vi "SmoothLine.vi"(8 "error in (no error)":errorcluster, 9 "Parameters":T2={"number of planes"=4, "z step"=1.9999999999999998e-05, "pixel dwell time"=1.0000000000000001e-11, "z frequency"=10.0, "number of pixels"=100, "smooth points"=10, "smooth line"=10, "Sine\nSawtooth"=FALSE, "PointSorting"=0, "Sort Points"=FALSE, "X-pixels"=256.0, "Y-lines"=256.0, "pixelstoµm"=256.0, "zoom"=1.0, "Time offset"=1.0000000000000001e-11} {"zoom" min=0.5 step=0.1; "Y-lines" min=1 step=1; "X-pixels" min=1 step=1; "PointSorting" items=["No Difference", "Every Second Point", "Down / Up"]; "smooth line" min=1; "smooth points" min=1; "number of pixels" min=1; "z frequency" format="%_4g"; "number of planes" min=1}, 10 "DutyCluster":T1 {"Iteration" items=["first iteration", "second iteration"]}, 11 "XYZ Point coordinates (pixels)":dbl[][](array[numeric])) -> (0 "error out":errorcluster, 2 "DutyCluster":T1 {"Iteration" items=["first iteration", "second iteration"]}, 3 "XYZ Point coordinates smoothed (pixels)":dbl[][](array[numeric]))   [LabVIEW 2010]
uses:
  TypeDefs/DutyCluster.ctl
  TypeDefs/ParameterCluster.ctl
  <vilib>/Analysis/_algsub.llb/Real Vector Norm.vi
  <vilib>/Analysis/NI_AALPro.lvlib
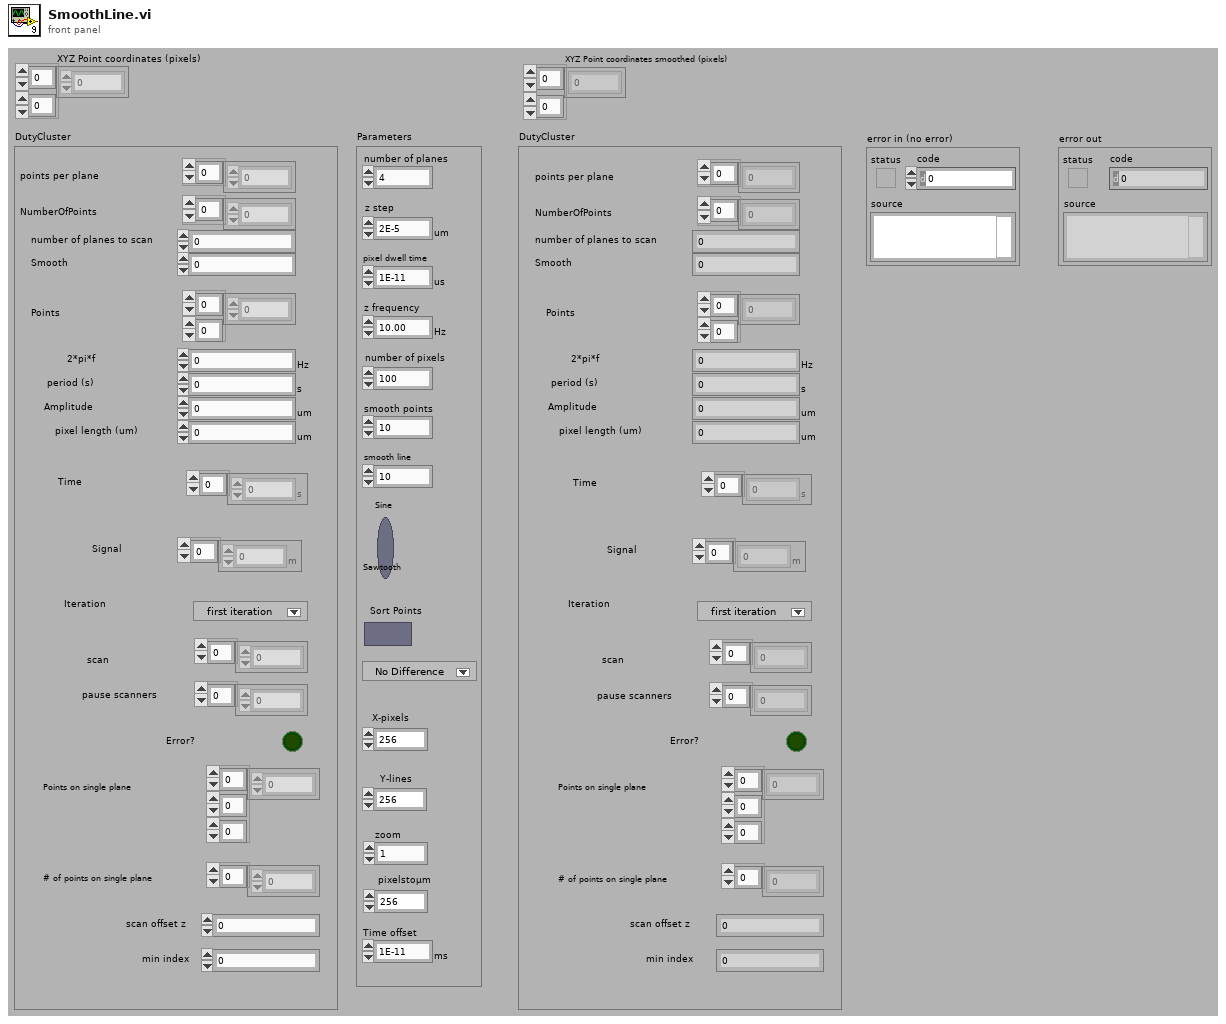
[diagram p1: front panel]
types:
  T1 = typedef "DutyCluster.ctl" = cluster{"points per plane":i32[], "NumberOfPoints":i32[], "number of planes to scan":i32, "Smooth":i32, "Points":dbl[][], "2*pi*f":dbl[unit], "period (s)":dbl[unit], "Amplitude":dbl[unit], "pixel length (um)":dbl[unit], "Time":dbl[unit][], "Signal":dbl[unit][], "Iteration":u16, "scan":i32[], "pause scanners":i32[], "Error?":bool, "Points on single plane":dbl[][][], "# of points on single plane":i32[], "scan offset z":i32, "min index":i32}
  T2 = typedef "ParameterCluster.ctl" = cluster{"number of planes":i32, "z step":dbl[unit], "pixel dwell time":dbl[unit], "z frequency":dbl[unit], "number of pixels":i32, "smooth points":i32, "smooth line":i32, "Sine\nSawtooth":bool, "PointSorting":u16, "Sort Points":bool, "X-pixels":sgl, "Y-lines":sgl, "pixelstoµm":dbl, "zoom":dbl, "Time offset":dbl[unit]}
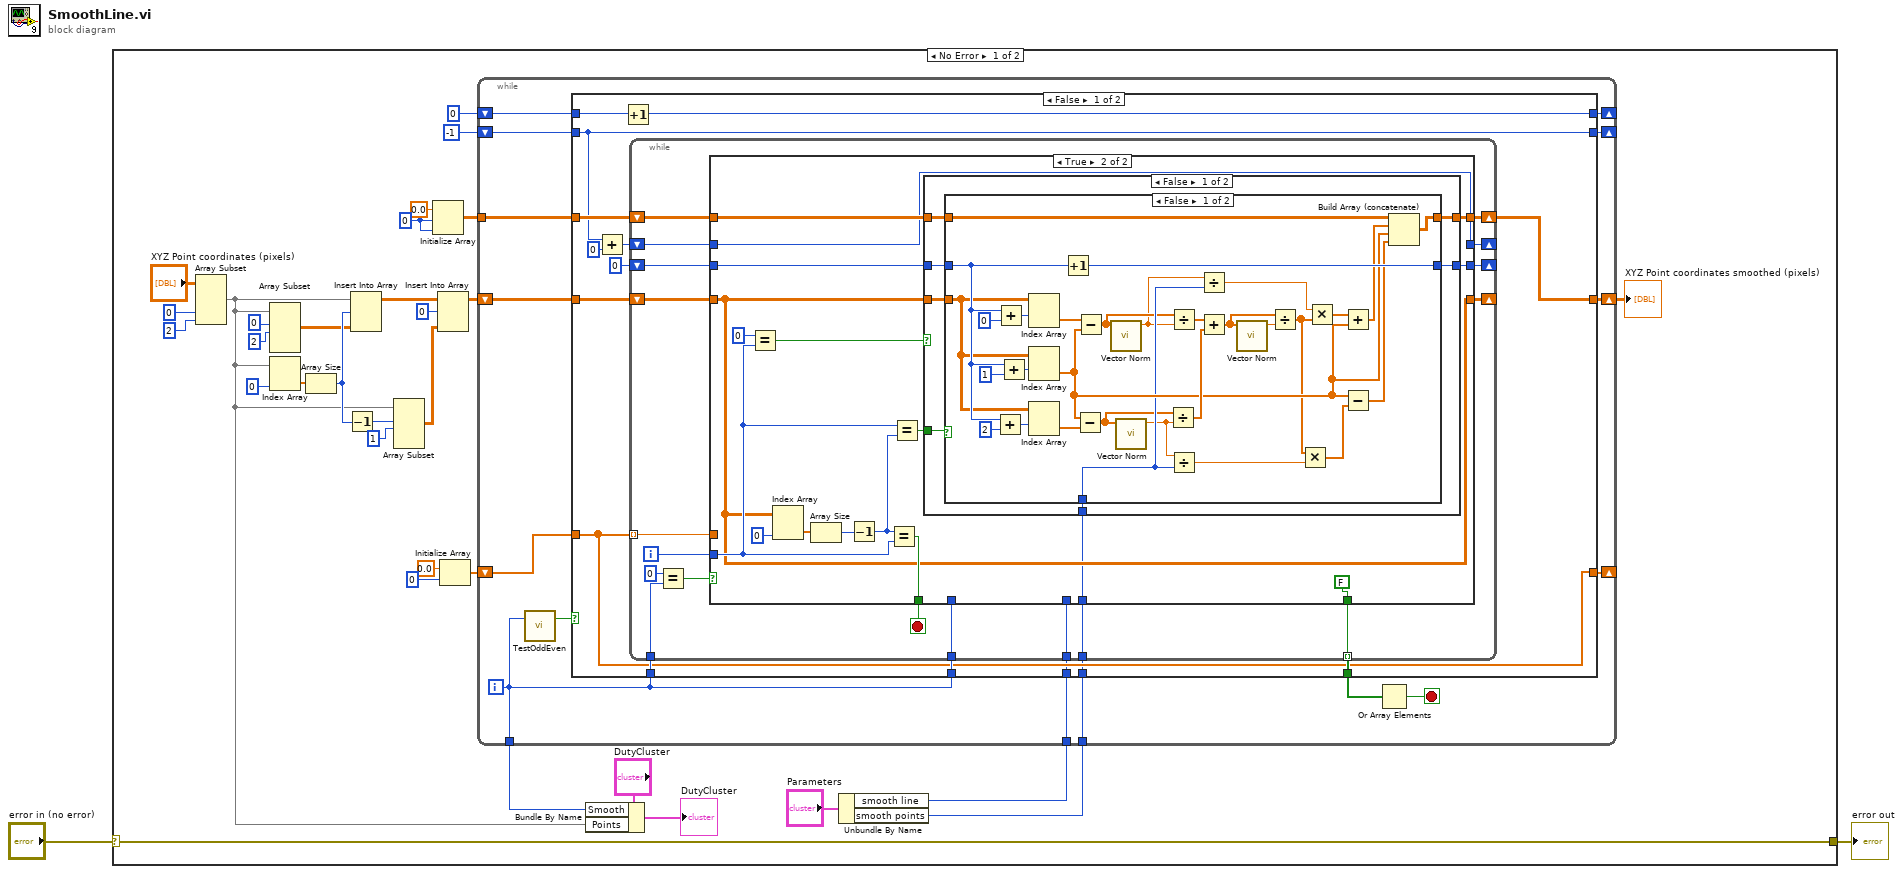
[diagram p0: block diagram]
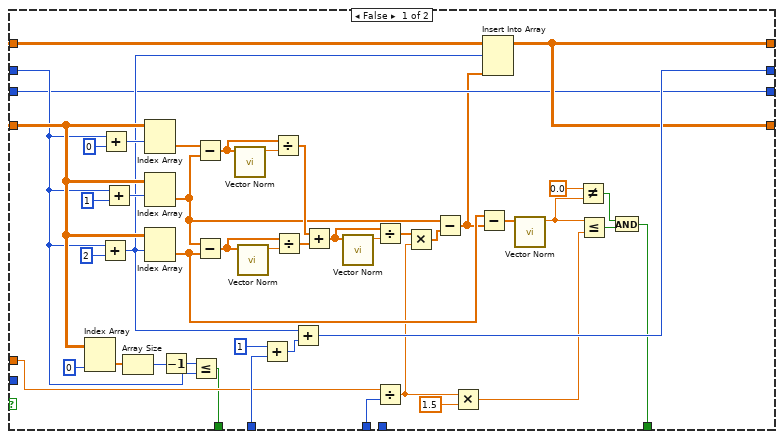
[diagram p2: hidden frame]
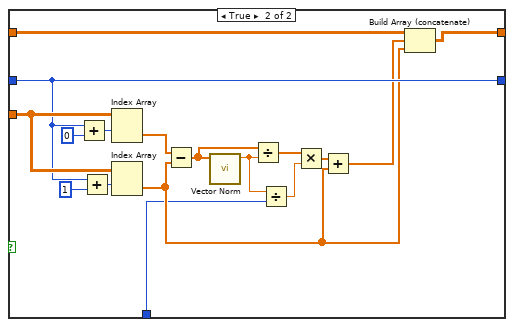
[diagram p3: hidden frame]
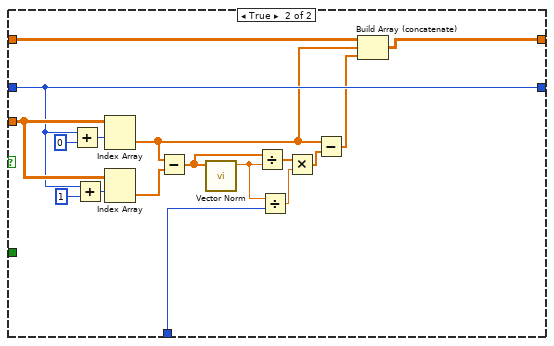
[diagram p4: hidden frame]
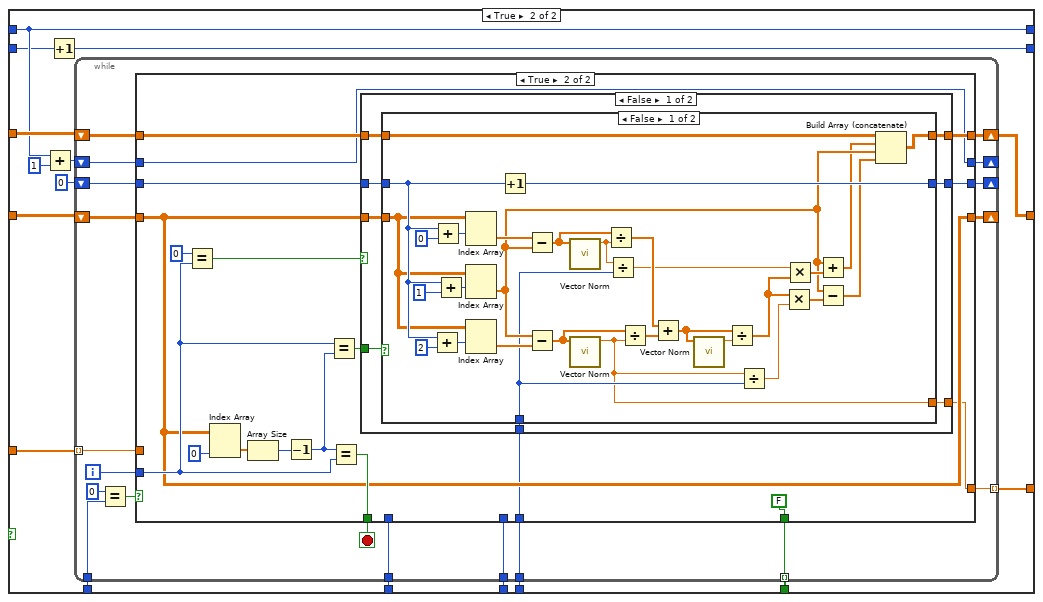
[diagram p5: hidden frame]
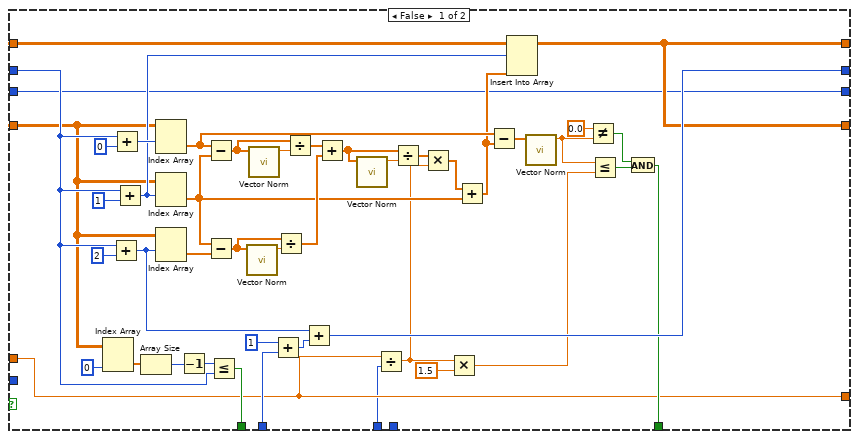
[diagram p6: hidden frame]
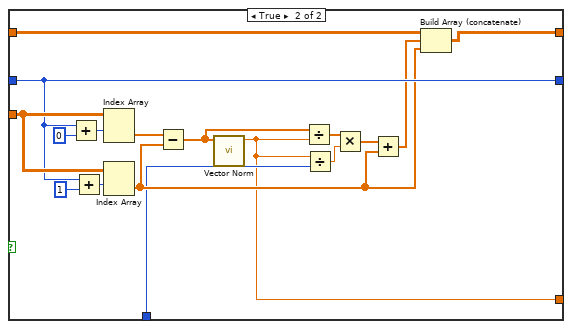
[diagram p7: hidden frame]
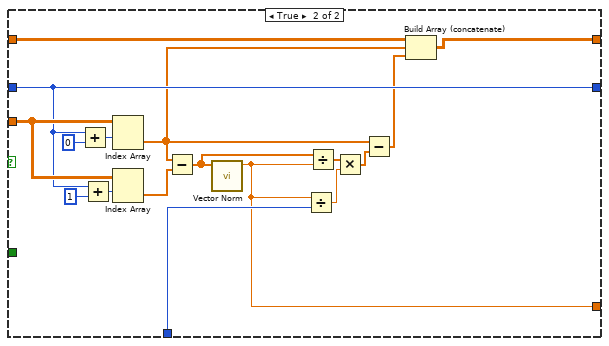
[diagram p8: hidden frame]
diagram:
  n1 = case shown="No Error" "error in (no error)" {
    selector: "error in (no error)" -> [w5 w384]
    tunnel: [w5 w384] -> w1
    frame No Error {
      w10 = 0 ("dimension size")
      n2 = Array Subset(array="XYZ Point coordinates (pixels)", index (col)=0 ("index"), length (col)=2 ("length")) -> (w9:dbl[][])  [unwired: 2 in]
      n3 = Array Subset(array=w9, index (row)=0 ("disabled index (col)"), length (row)=2 ("length")) -> (w17:dbl[][])  [unwired: 2 in]
      n4 = Index Array(array=w9, index (col)=0 ("disabled index (col)")) -> (element=w15:dbl[])  [unwired: 1 in]
      n5 = Array Size(array=w15) -> (size(s)=w18:i32)
      n6 = Decrement(x=w18) -> (x-1=w24:i32)
      n7 = Insert Into Array(array=w9, index (row)=w18, new element=w17) -> (w21:dbl[][])  [unwired: 1 in]
      n8 = Array Subset(array=w9, index (row)=w24, length (row)=1 ("length")) -> (w19:dbl[][])  [unwired: 2 in]
      n9 = Initialize Array(0.0 ("element"), w10, w10) -> (w33:dbl[][])
      n10 = Insert Into Array(array=w21, index (row)=0, new element=w19) -> (w27:dbl[][])  [unwired: 1 in]
      n11 = Initialize Array(0.0 ("element"), 0 ("dimension size")) -> (w28:dbl[])
      n12 = Unbundle By Name("Parameters") -> ("smooth line"=w8:i32, "smooth points"=w7:i32)
      n13 = while {
        shift-right: [w47] -> w6
        shift-left: w27 -> [w49]
        tunnel: w33 -> [w48]
        shift-right: [w43] -> _
        shift-left: 0 ("index") -> [w44]
        shift-right: [w41] -> _
        shift-left: -1 ("index") -> [w42]
        tunnel: [w40] -> w12
        shift-right: [w39] -> _
        shift-left: w28 -> [w38]
        tunnel: w8 -> [w36]
        tunnel: w7 -> [w35]
        i -> [w40]
        stop <- w37 stop-if-true
        n14 = call "TestOddEven.vi"("Numeric"=w40) -> ("Boolean"=w45:bool)  [unwired: 1 in, 1 out]
        n15 = case shown="False" w45 {
          tunnel: w49 -> [w63 w229]
          tunnel: w48 -> [w62 w230]
          tunnel: [w61 w224] -> w47
          tunnel: [w60 w228] -> w46
          tunnel: w40 -> [w59 w227]
          tunnel: w40 -> [w58 w226]
          tunnel: w44 -> [w57 w221]
          tunnel: [w56 w221] -> w43
          tunnel: w42 -> [w55 w220]
          tunnel: [w55 w219] -> w41
          tunnel: [w52 w218] -> w39
          tunnel: w38 -> [w52 w217]
          tunnel: w36 -> [w51 w216]
          tunnel: w35 -> [w50 w215]
          frame False {
            n16 = Add(x=w55, y=0) -> (x+y=w54:i32)
            n17 = Increment(x=w57) -> (x+1=w56:i32)
            n18 = while {
              shift-right: [w82] -> _
              shift-left: 0 ("index") -> [w78]
              shift-right: [w80] -> w61
              shift-left: w62 -> [w81]
              tunnel: w59 -> [w71]
              shift-right: [w75] -> _
              shift-left: w54 -> [w70]
              shift-right: [w74] -> _
              shift-left: w63 -> [w79]
              tunnel: w58 -> [w73]
              tunnel: [w72] -> w60 mode=indexing
              tunnel: w52 -> [w68] mode=indexing
              tunnel: w51 -> [w66]
              tunnel: w50 -> [w65]
              i -> [w69]
              stop <- w67 stop-if-true
              n19 = Equal?(x=0 ("y"), y=w71) -> (x = y?=w76:bool)
              n20 = case shown="True" w76 {
                tunnel: [w99 w143] -> w82
                tunnel: [w92 w142] -> w67
                tunnel: w81 -> [_ w141]
                tunnel: [w115 w140] -> w80
                tunnel: w79 -> [w105 w129]
                tunnel: w78 -> [w99 w137]
                tunnel: w69 -> [_ w133]
                tunnel: w70 -> [w101 w130]
                tunnel: [w116 w130] -> w75
                tunnel: [w115 w129] -> w74
                tunnel: w73 -> [w111 _]
                tunnel: [w109 FALSE] -> w72
                tunnel: w68 -> [w94 _]
                tunnel: w66 -> [w91 _]
                tunnel: w65 -> [_ w127]
                frame False {
                  n21 = Index Array(array=w105, index (col)=0 ("disabled index (col)")) -> (element=w126:dbl[])  [unwired: 1 in]
                  n22 = Add(x=w101, y=2 ("disabled index (col)")) -> (x+y=w104:i32)
                  n23 = Add(x=w101, y=0 ("disabled index (col)")) -> (x+y=w121:i32)
                  n24 = Add(x=w101, y=1 ("disabled index (col)")) -> (x+y=w114:i32)
                  n25 = Array Size(array=w126) -> (size(s)=w124:i32)
                  n26 = Index Array(array=w105, index (row)=w121) -> (element=w108:dbl[])  [unwired: 1 in]
                  n27 = Index Array(array=w105, index (row)=w114) -> (element=w102:dbl[])  [unwired: 1 in]
                  n28 = Index Array(array=w105, index (row)=w104) -> (element=w100:dbl[])  [unwired: 1 in]
                  n29 = Decrement(x=w124) -> (x-1=w123:i32)
                  n30 = Less Or Equal?(x=w123, y=w101) -> (x <= y?=w92:bool)
                  n31 = Subtract(x=w108, y=w102) -> (x-y=w90:dbl[])
                  n32 = Subtract(x=w102, y=w100) -> (x-y=w88:dbl[])
                  n33 = call-poly <vilib>:"Vector Norm.vi"("Input Vector"=w90) -> ("norm"=w89:dbl)  [unwired: 9 in, 1 out]
                  n34 = call-poly <vilib>:"Vector Norm.vi"("Input Vector"=w88) -> ("norm"=w87:dbl)  [unwired: 9 in, 1 out]
                  n35 = Add(x=1 ("y"), y=w111) -> (x+y=w113:i32)
                  n36 = Divide(x=w90, y=w89) -> (x/y=w118:dbl[])
                  n37 = Divide(x=w88, y=w87) -> (x/y=w117:dbl[])
                  n38 = Add(x=w104, y=w113) -> (x+y=w116:i32)
                  n39 = Add(x=w118, y=w117) -> (x+y=w86:dbl[])
                  n40 = call-poly <vilib>:"Vector Norm.vi"("Input Vector"=w86) -> ("norm"=w85:dbl)  [unwired: 9 in, 1 out]
                  n41 = Divide(x=w86, y=w85) -> (x/y=w97:dbl[])
                  n42 = Divide(x=w94, y=w91) -> (x/y=w93:dbl)
                  n43 = Multiply(x=w97, y=w93) -> (x*y=w103:dbl[])
                  n44 = Subtract(x=w102, y=w103) -> (x-y=w98:dbl[])
                  n45 = Multiply(x=w93, y=1.5) -> (x*y=w95:dbl)
                  n46 = Subtract(x=w100, y=w98) -> (x-y=w84:dbl[])
                  n47 = Insert Into Array(array=w105, index (row)=w104, new element=w98) -> (w115:dbl[][])  [unwired: 1 in]
                  n48 = call-poly <vilib>:"Vector Norm.vi"("Input Vector"=w84) -> ("norm"=w83:dbl)  [unwired: 9 in, 1 out]
                  n49 = Not Equal?(x=0.0, y=w83) -> (x != y?=w107:bool)
                  n50 = Less Or Equal?(x=w83, y=w95) -> (x <= y?=w110:bool)
                  n51 = And(x=w107, y=w110) -> (x .and. y?=w109:bool)
                }
                frame True {
                  n52 = Equal?(x=0 ("y"), y=w133) -> (x = y?=w136:bool)
                  n53 = Index Array(array=w129, index (col)=0 ("disabled index (col)")) -> (element=w139:dbl[])  [unwired: 1 in]
                  n54 = Array Size(array=w139) -> (size(s)=w132:i32)
                  n55 = Decrement(x=w132) -> (x-1=w131:i32)
                  n56 = Equal?(x=w131, y=w133) -> (x = y?=w142:bool)
                  n57 = Equal?(x=w133, y=w131) -> (x = y?=w134:bool)
                  n58 = case shown="False" w136 {
                    tunnel: [w150 w211] -> w143
                    tunnel: w137 -> [w149 w211]
                    tunnel: w141 -> [w148 w213]
                    tunnel: [w147 w212] -> w140
                    tunnel: w129 -> [w146 w214]
                    tunnel: w134 -> [w145 _]
                    tunnel: w127 -> [w144 w200]
                    frame False {
                      n59 = case shown="False" w145 {
                        tunnel: [w174 w189] -> w150
                        tunnel: w149 -> [w173 w189]
                        tunnel: w148 -> [w172 w192]
                        tunnel: [w166 w191] -> w147
                        tunnel: w146 -> [w165 w190]
                        tunnel: w144 -> [w157 w183]
                        frame False {
                          n60 = Add(x=w173, y=2 ("disabled index (col)")) -> (x+y=w175:i32)
                          n61 = Add(x=w173, y=0 ("disabled index (col)")) -> (x+y=w179:i32)
                          n62 = Add(x=w173, y=1 ("disabled index (col)")) -> (x+y=w177:i32)
                          n63 = Index Array(array=w165, index (row)=w179) -> (element=w170:dbl[])  [unwired: 1 in]
                          n64 = Index Array(array=w165, index (row)=w177) -> (element=w164:dbl[])  [unwired: 1 in]
                          n65 = Index Array(array=w165, index (row)=w175) -> (element=w171:dbl[])  [unwired: 1 in]
                          n66 = Increment(x=w173) -> (x+1=w174:i32)
                          n67 = Subtract(x=w164, y=w171) -> (x-y=w154:dbl[])
                          n68 = Subtract(x=w170, y=w164) -> (x-y=w156:dbl[])
                          n69 = call-poly <vilib>:"Vector Norm.vi"("Input Vector"=w156) -> ("norm"=w155:dbl)  [unwired: 9 in, 1 out]
                          n70 = call-poly <vilib>:"Vector Norm.vi"("Input Vector"=w154) -> ("norm"=w153:dbl)  [unwired: 9 in, 1 out]
                          n71 = Divide(x=w154, y=w153) -> (x/y=w168:dbl[])
                          n72 = Divide(x=w156, y=w155) -> (x/y=w169:dbl[])
                          n73 = Divide(x=w153, y=w157) -> (x/y=w159:dbl)
                          n74 = Divide(x=w155, y=w157) -> (x/y=w158:dbl)
                          n75 = Add(x=w169, y=w168) -> (x+y=w152:dbl[])
                          n76 = call-poly <vilib>:"Vector Norm.vi"("Input Vector"=w152) -> ("norm"=w151:dbl)  [unwired: 9 in, 1 out]
                          n77 = Divide(x=w152, y=w151) -> (x/y=w161:dbl[])
                          n78 = Multiply(x=w161, y=w159) -> (x*y=w160:dbl[])
                          n79 = Multiply(x=w158, y=w161) -> (x*y=w167:dbl[])
                          n80 = Add(x=w167, y=w164) -> (x+y=w162:dbl[])
                          n81 = Subtract(x=w164, y=w160) -> (x-y=w163:dbl[])
                          n82 = Build Array (concatenate)(w172, w162, w164, w163) -> (w166:dbl[][])
                        }
                        frame True {
                          n83 = Add(x=w189, y=0 ("disabled index (col)")) -> (x+y=w196:i32)
                          n84 = Add(x=w189, y=1 ("disabled index (col)")) -> (x+y=w194:i32)
                          n85 = Index Array(array=w190, index (row)=w196) -> (element=w193:dbl[])  [unwired: 1 in]
                          n86 = Index Array(array=w190, index (row)=w194) -> (element=w187:dbl[])  [unwired: 1 in]
                          n87 = Subtract(x=w193, y=w187) -> (x-y=w182:dbl[])
                          n88 = call-poly <vilib>:"Vector Norm.vi"("Input Vector"=w182) -> ("norm"=w181:dbl)  [unwired: 9 in, 1 out]
                          n89 = Divide(x=w182, y=w181) -> (x/y=w185:dbl[])
                          n90 = Divide(x=w181, y=w183) -> (x/y=w184:dbl)
                          n91 = Multiply(x=w185, y=w184) -> (x*y=w188:dbl[])
                          n92 = Add(x=w188, y=w187) -> (x+y=w186:dbl[])
                          n93 = Build Array (concatenate)(w192, w186, w187) -> (w191:dbl[][])
                        }
                      }
                    }
                    frame True {
                      n94 = Add(x=w211, y=0 ("disabled index (col)")) -> (x+y=w209:i32)
                      n95 = Add(x=w211, y=1 ("disabled index (col)")) -> (x+y=w207:i32)
                      n96 = Index Array(array=w214, index (row)=w209) -> (element=w206:dbl[])  [unwired: 1 in]
                      n97 = Index Array(array=w214, index (row)=w207) -> (element=w205:dbl[])  [unwired: 1 in]
                      n98 = Subtract(x=w206, y=w205) -> (x-y=w199:dbl[])
                      n99 = call-poly <vilib>:"Vector Norm.vi"("Input Vector"=w199) -> ("norm"=w198:dbl)  [unwired: 9 in, 1 out]
                      n100 = Divide(x=w199, y=w198) -> (x/y=w203:dbl[])
                      n101 = Divide(x=w198, y=w200) -> (x/y=w201:dbl)
                      n102 = Multiply(x=w203, y=w201) -> (x*y=w204:dbl[])
                      n103 = Subtract(x=w206, y=w204) -> (x-y=w202:dbl[])
                      n104 = Build Array (concatenate)(w213, w206, w202) -> (w212:dbl[][])
                    }
                  }
                }
              }
            }
          }
          frame True {
            n105 = Add(x=w221, y=1 ("index")) -> (x+y=w222:i32)
            n106 = Increment(x=w220) -> (x+1=w219:i32)
            n107 = while {
              shift-right: [w249] -> _
              shift-left: 0 ("index") -> [w245]
              shift-right: [w247] -> w224
              shift-left: w230 -> [w248]
              tunnel: w227 -> [w242]
              shift-right: [w239] -> _
              shift-left: w222 -> [w240]
              shift-right: [w238] -> _
              shift-left: w229 -> [w246]
              tunnel: w226 -> [w237]
              tunnel: [w236] -> w228 mode=indexing
              tunnel: [w235] -> w218 mode=indexing
              tunnel: w217 -> [w234] mode=indexing
              tunnel: w216 -> [w232]
              tunnel: w215 -> [w231]
              i -> [w244]
              stop <- w233 stop-if-true
              n108 = Equal?(x=0 ("y"), y=w242) -> (x = y?=w241:bool)
              n109 = case shown="True" w241 {
                tunnel: [w264 w311] -> w249
                tunnel: [w290 w310] -> w233
                tunnel: w248 -> [_ w309]
                tunnel: [w279 w308] -> w247
                tunnel: w246 -> [w268 w297]
                tunnel: w245 -> [w264 w305]
                tunnel: w244 -> [_ w301]
                tunnel: w240 -> [w281 w298]
                tunnel: [w280 w298] -> w239
                tunnel: [w279 w297] -> w238
                tunnel: w237 -> [w274 _]
                tunnel: [w272 FALSE] -> w236
                tunnel: [w260 w295] -> w235
                tunnel: w234 -> [w260 _]
                tunnel: w232 -> [w258 _]
                tunnel: w231 -> [_ w294]
                frame False {
                  n110 = Index Array(array=w268, index (col)=0 ("disabled index (col)")) -> (element=w293:dbl[])  [unwired: 1 in]
                  n111 = Add(x=w281, y=2 ("disabled index (col)")) -> (x+y=w277:i32)
                  n112 = Add(x=w281, y=0 ("disabled index (col)")) -> (x+y=w287:i32)
                  n113 = Add(x=w281, y=1 ("disabled index (col)")) -> (x+y=w278:i32)
                  n114 = Array Size(array=w293) -> (size(s)=w291:i32)
                  n115 = Index Array(array=w268, index (row)=w287) -> (element=w271:dbl[])  [unwired: 1 in]
                  n116 = Index Array(array=w268, index (row)=w278) -> (element=w265:dbl[])  [unwired: 1 in]
                  n117 = Index Array(array=w268, index (row)=w277) -> (element=w284:dbl[])  [unwired: 1 in]
                  n118 = Decrement(x=w291) -> (x-1=w289:i32)
                  n119 = Subtract(x=w271, y=w265) -> (x-y=w255:dbl[])
                  n120 = Subtract(x=w265, y=w284) -> (x-y=w257:dbl[])
                  n121 = Less Or Equal?(x=w289, y=w281) -> (x <= y?=w290:bool)
                  n122 = call-poly <vilib>:"Vector Norm.vi"("Input Vector"=w257) -> ("norm"=w256:dbl)  [unwired: 9 in, 1 out]
                  n123 = call-poly <vilib>:"Vector Norm.vi"("Input Vector"=w255) -> ("norm"=w254:dbl)  [unwired: 9 in, 1 out]
                  n124 = Add(x=1 ("y"), y=w274) -> (x+y=w276:i32)
                  n125 = Divide(x=w257, y=w256) -> (x/y=w282:dbl[])
                  n126 = Divide(x=w255, y=w254) -> (x/y=w283:dbl[])
                  n127 = Add(x=w277, y=w276) -> (x+y=w280:i32)
                  n128 = Add(x=w283, y=w282) -> (x+y=w253:dbl[])
                  n129 = call-poly <vilib>:"Vector Norm.vi"("Input Vector"=w253) -> ("norm"=w252:dbl)  [unwired: 9 in, 1 out]
                  n130 = Divide(x=w260, y=w258) -> (x/y=w259:dbl)
                  n131 = Divide(x=w253, y=w252) -> (x/y=w263:dbl[])
                  n132 = Multiply(x=w263, y=w259) -> (x*y=w266:dbl[])
                  n133 = Multiply(x=w259, y=1.5) -> (x*y=w261:dbl)
                  n134 = Add(x=w266, y=w265) -> (x+y=w267:dbl[])
                  n135 = Subtract(x=w271, y=w267) -> (x-y=w251:dbl[])
                  n136 = Insert Into Array(array=w268, index (row)=w278, new element=w267) -> (w279:dbl[][])  [unwired: 1 in]
                  n137 = call-poly <vilib>:"Vector Norm.vi"("Input Vector"=w251) -> ("norm"=w250:dbl)  [unwired: 9 in, 1 out]
                  n138 = Not Equal?(x=0.0, y=w250) -> (x != y?=w270:bool)
                  n139 = Less Or Equal?(x=w250, y=w261) -> (x <= y?=w273:bool)
                  n140 = And(x=w270, y=w273) -> (x .and. y?=w272:bool)
                }
                frame True {
                  n141 = Equal?(x=0 ("y"), y=w301) -> (x = y?=w304:bool)
                  n142 = Index Array(array=w297, index (col)=0 ("disabled index (col)")) -> (element=w307:dbl[])  [unwired: 1 in]
                  n143 = Array Size(array=w307) -> (size(s)=w300:i32)
                  n144 = Decrement(x=w300) -> (x-1=w299:i32)
                  n145 = Equal?(x=w301, y=w299) -> (x = y?=w302:bool)
                  n146 = Equal?(x=w299, y=w301) -> (x = y?=w310:bool)
                  n147 = case shown="False" w304 {
                    tunnel: [w319 w380] -> w311
                    tunnel: w305 -> [w318 w380]
                    tunnel: w309 -> [w317 w382]
                    tunnel: [w316 w381] -> w308
                    tunnel: w297 -> [w315 w383]
                    tunnel: w302 -> [w314 _]
                    tunnel: [w313 w367] -> w295
                    tunnel: w294 -> [w312 w369]
                    frame False {
                      n148 = case shown="False" w314 {
                        tunnel: [w343 w358] -> w319
                        tunnel: w318 -> [w342 w358]
                        tunnel: w317 -> [w341 w361]
                        tunnel: [w336 w360] -> w316
                        tunnel: w315 -> [w335 w359]
                        tunnel: [w322 w350] -> w313
                        tunnel: w312 -> [w326 w352]
                        frame False {
                          n149 = Add(x=w342, y=2 ("disabled index (col)")) -> (x+y=w344:i32)
                          n150 = Add(x=w342, y=0 ("disabled index (col)")) -> (x+y=w348:i32)
                          n151 = Add(x=w342, y=1 ("disabled index (col)")) -> (x+y=w346:i32)
                          n152 = Index Array(array=w335, index (row)=w348) -> (element=w339:dbl[])  [unwired: 1 in]
                          n153 = Index Array(array=w335, index (row)=w346) -> (element=w329:dbl[])  [unwired: 1 in]
                          n154 = Index Array(array=w335, index (row)=w344) -> (element=w340:dbl[])  [unwired: 1 in]
                          n155 = Increment(x=w342) -> (x+1=w343:i32)
                          n156 = Subtract(x=w339, y=w329) -> (x-y=w325:dbl[])
                          n157 = Subtract(x=w329, y=w340) -> (x-y=w323:dbl[])
                          n158 = call-poly <vilib>:"Vector Norm.vi"("Input Vector"=w325) -> ("norm"=w324:dbl)  [unwired: 9 in, 1 out]
                          n159 = call-poly <vilib>:"Vector Norm.vi"("Input Vector"=w323) -> ("norm"=w322:dbl)  [unwired: 9 in, 1 out]
                          n160 = Divide(x=w325, y=w324) -> (x/y=w338:dbl[])
                          n161 = Divide(x=w324, y=w326) -> (x/y=w332:dbl)
                          n162 = Divide(x=w323, y=w322) -> (x/y=w337:dbl[])
                          n163 = Add(x=w338, y=w337) -> (x+y=w321:dbl[])
                          n164 = call-poly <vilib>:"Vector Norm.vi"("Input Vector"=w321) -> ("norm"=w320:dbl)  [unwired: 9 in, 1 out]
                          n165 = Divide(x=w321, y=w320) -> (x/y=w333:dbl[])
                          n166 = Divide(x=w322, y=w326) -> (x/y=w334:dbl)
                          n167 = Multiply(x=w333, y=w334) -> (x*y=w330:dbl[])
                          n168 = Multiply(x=w332, y=w333) -> (x*y=w331:dbl[])
                          n169 = Add(x=w329, y=w331) -> (x+y=w328:dbl[])
                          n170 = Subtract(x=w329, y=w330) -> (x-y=w327:dbl[])
                          n171 = Build Array (concatenate)(w341, w328, w329, w327) -> (w336:dbl[][])
                        }
                        frame True {
                          n172 = Add(x=w358, y=0 ("disabled index (col)")) -> (x+y=w365:i32)
                          n173 = Add(x=w358, y=1 ("disabled index (col)")) -> (x+y=w363:i32)
                          n174 = Index Array(array=w359, index (row)=w365) -> (element=w362:dbl[])  [unwired: 1 in]
                          n175 = Index Array(array=w359, index (row)=w363) -> (element=w356:dbl[])  [unwired: 1 in]
                          n176 = Subtract(x=w362, y=w356) -> (x-y=w351:dbl[])
                          n177 = call-poly <vilib>:"Vector Norm.vi"("Input Vector"=w351) -> ("norm"=w350:dbl)  [unwired: 9 in, 1 out]
                          n178 = Divide(x=w351, y=w350) -> (x/y=w354:dbl[])
                          n179 = Divide(x=w350, y=w352) -> (x/y=w353:dbl)
                          n180 = Multiply(x=w354, y=w353) -> (x*y=w357:dbl[])
                          n181 = Add(x=w357, y=w356) -> (x+y=w355:dbl[])
                          n182 = Build Array (concatenate)(w361, w355, w356) -> (w360:dbl[][])
                        }
                      }
                    }
                    frame True {
                      n183 = Add(x=w380, y=0 ("disabled index (col)")) -> (x+y=w378:i32)
                      n184 = Add(x=w380, y=1 ("disabled index (col)")) -> (x+y=w376:i32)
                      n185 = Index Array(array=w383, index (row)=w378) -> (element=w375:dbl[])  [unwired: 1 in]
                      n186 = Index Array(array=w383, index (row)=w376) -> (element=w374:dbl[])  [unwired: 1 in]
                      n187 = Subtract(x=w375, y=w374) -> (x-y=w368:dbl[])
                      n188 = call-poly <vilib>:"Vector Norm.vi"("Input Vector"=w368) -> ("norm"=w367:dbl)  [unwired: 9 in, 1 out]
                      n189 = Divide(x=w367, y=w369) -> (x/y=w370:dbl)
                      n190 = Divide(x=w368, y=w367) -> (x/y=w372:dbl[])
                      n191 = Multiply(x=w372, y=w370) -> (x*y=w373:dbl[])
                      n192 = Subtract(x=w375, y=w373) -> (x-y=w371:dbl[])
                      n193 = Build Array (concatenate)(w382, w375, w371) -> (w381:dbl[][])
                    }
                  }
                }
              }
            }
          }
        }
        n194 = Or Array Elements(Boolean array=w46) -> (logical OR=w37:bool)
      }
      "XYZ Point coordinates smoothed (pixels)" <- w6
      n195 = Bundle By Name(cluster="DutyCluster", "Smooth"=w12, "Points"=w9) -> (→"DutyCluster":T1)
    }
    frame Error {
    }
  }
  "error out" <- w1
